vi "Pull_Data_via_Public_Client.vi"(3 "application reference":refnum<vi>, 4 "error in (no error)":errorcluster, 5 "Archive Files?":bool, 6 "Running on Server?":bool, 7 "Path of File relative to EnFlo Data Root":path[](array[path])) -> (0 "error out":errorcluster, 1 "Error String":string)   [LabVIEW 2016]
uses:
  Anemometry/Anemometry Sub Vis/Globals/Constants_global.vi
  Sub VIs/Harvest_Global.vi
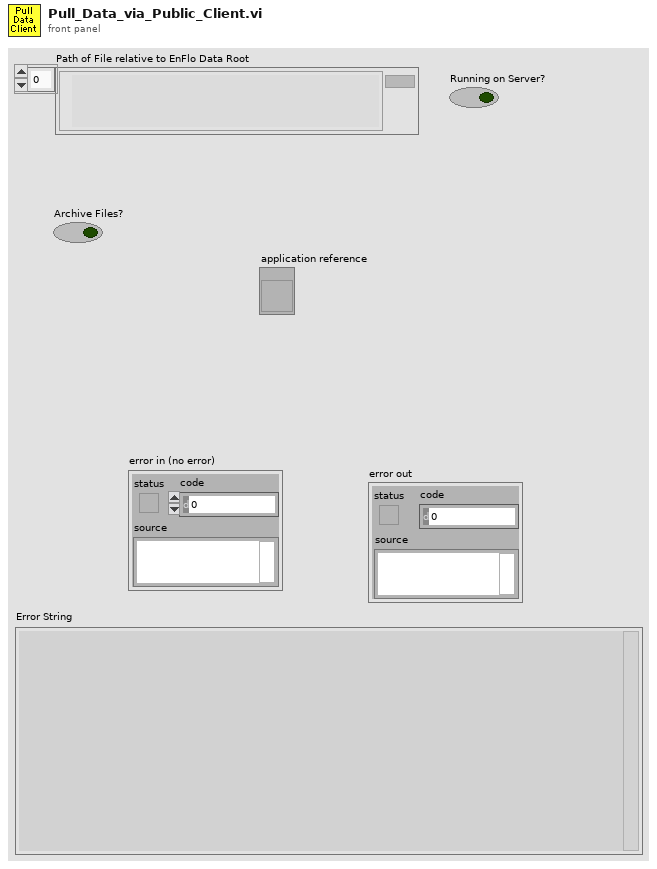
[diagram p1: front panel]
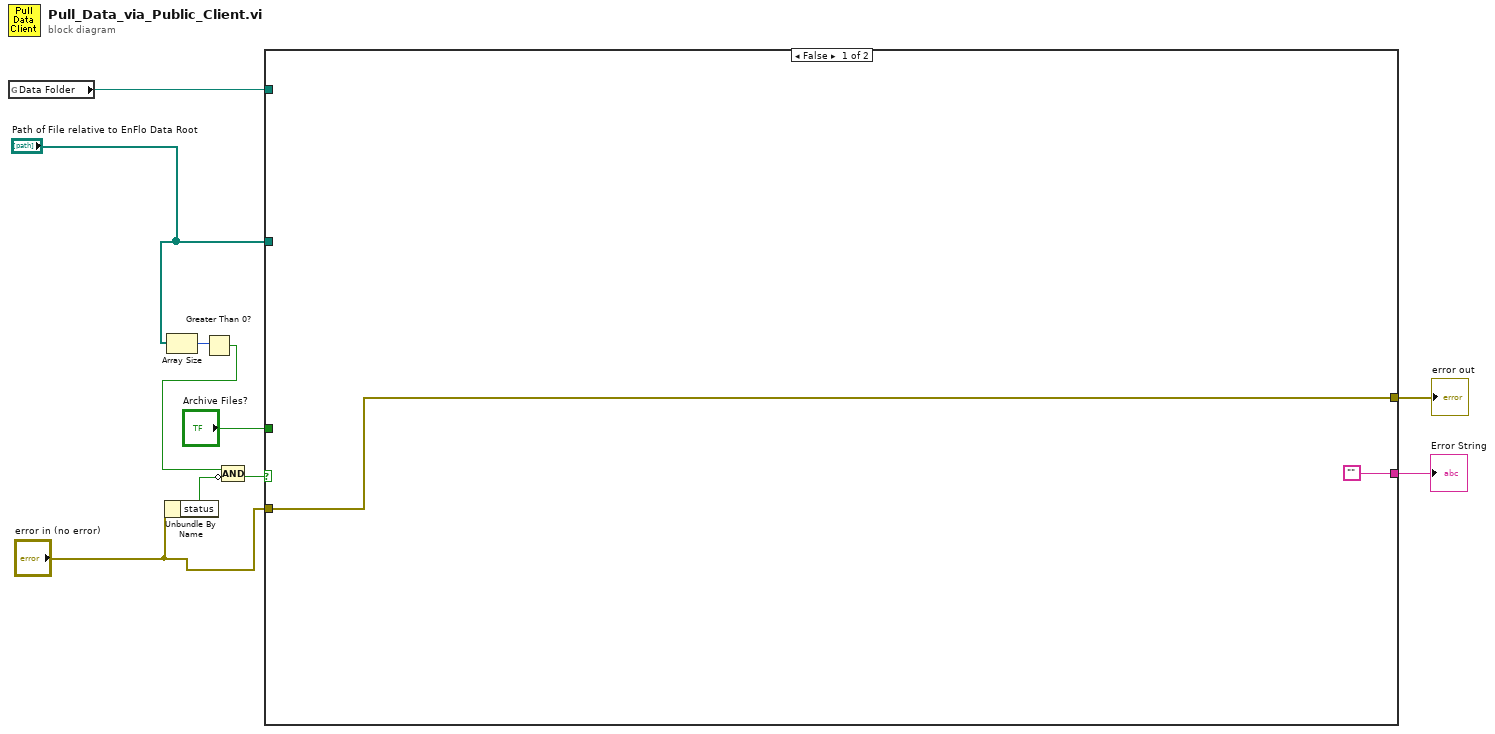
[diagram p0: block diagram]
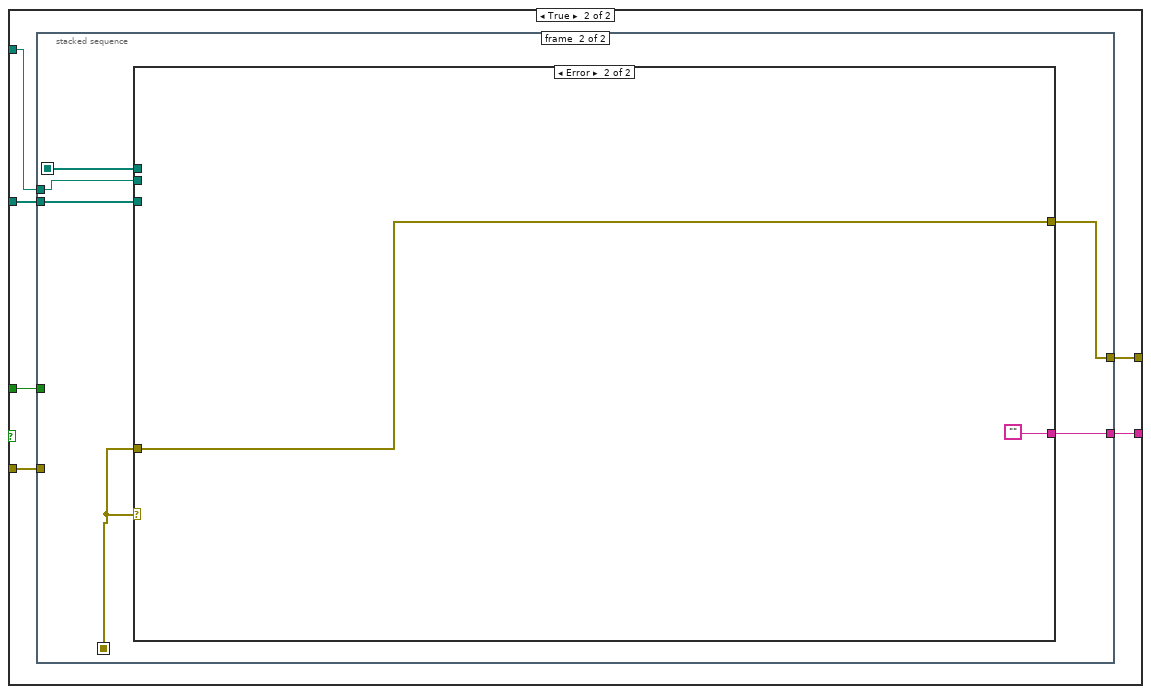
[diagram p2: hidden frame]
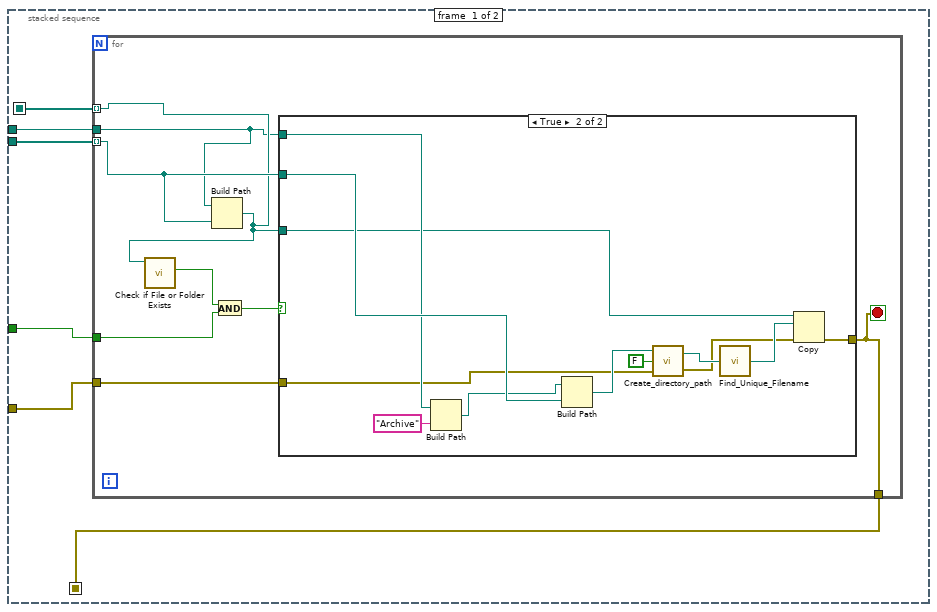
[diagram p3: hidden frame]
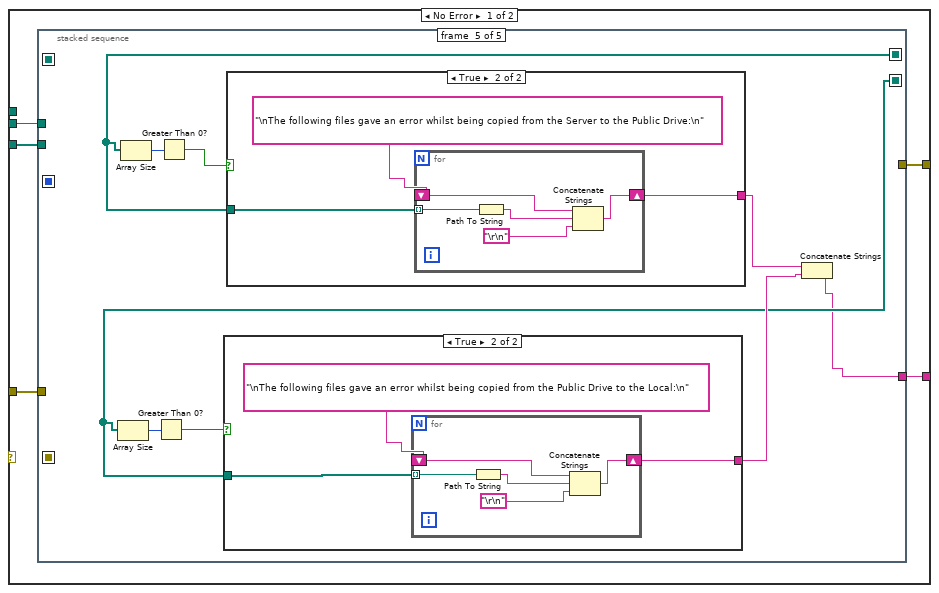
[diagram p5: hidden frame]
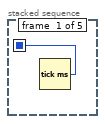
[diagram p6: hidden frame]
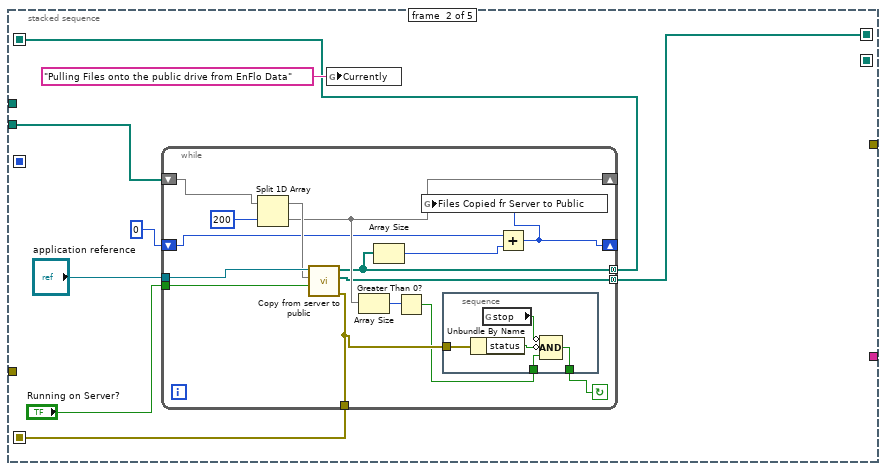
[diagram p7: hidden frame]
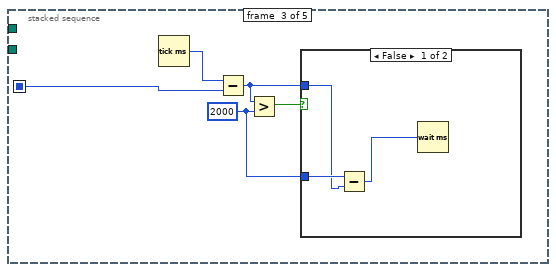
[diagram p8: hidden frame]
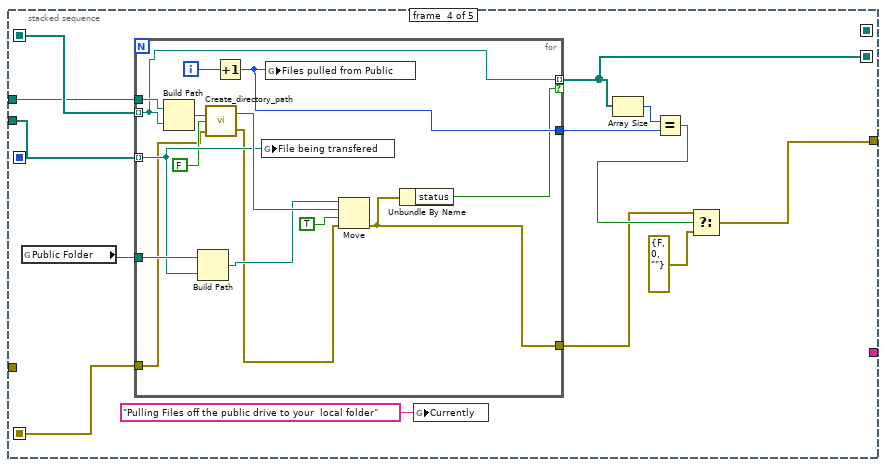
[diagram p10: hidden frame]
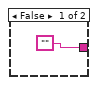
[diagram p11: hidden frame]
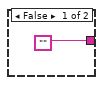
[diagram p12: hidden frame]
diagram:
  n1 = global read "Constants_global.vi" "Data Folder"() -> (w8:path)
  n2 = Unbundle By Name("error in (no error)") -> ("status"=w7:bool)
  n3 = Array Size(array="Path of File relative to EnFlo Data Root") -> (size(s)=w6:i32)
  n4 = Greater Than 0?(x=w6) -> (x > 0?=w5:bool)
  n5 = Compound Arithmetic op=AND(w5, invert w7) -> (w3:bool)
  n6 = case shown="False" w3 {
    tunnel: [w12 w18] -> w10
    tunnel: "error in (no error)" -> [w12 w17]
    tunnel: "Path of File relative to EnFlo Data Root" -> [_ w16]
    tunnel: "Archive Files?" -> [_ w15]
    tunnel: w8 -> [_ w14]
    tunnel: ["" w13] -> w1
    frame False {
    }
    frame True {
      n7 = stacked-sequence {
        seq-local: [w23 _] -> [_ w48]
        seq-local: [w21 _] -> [_ w50]
        tunnel: [_ w51] -> w18
        tunnel: w17 -> [w24 _]
        tunnel: w16 -> [w22 w49]
        tunnel: w15 -> [w20 _]
        tunnel: w14 -> [w19 w47]
        tunnel: [_ w46] -> w13
        frame #0 {
          n8 = for {
            tunnel: w24 -> [w32]
            tunnel: [w27] -> w23
            tunnel: w22 -> [w31] mode=indexing
            tunnel: w20 -> [w30]
            tunnel: [w26] -> w21 mode=indexing
            tunnel: w19 -> [w25]
            stop <- w27 stop-if-true
            n9 = Build Path(base path=w25, name or relative path=w31) -> (appended path=w26:path)
            n10 = call <vilib>:"Check if File or Folder Exists.vi"("path"=w26) -> ("file or folder exists?"=w29:bool)  [unwired: 8 in, 2 out]
            n11 = And(x=w29, y=w30) -> (x .and. y?=w28:bool)
            n12 = case shown="True" w28 {
              tunnel: w25 -> [_ w39]
              tunnel: w31 -> [_ w41]
              tunnel: [w33 w37] -> w27
              tunnel: w32 -> [w33 w36]
              tunnel: w26 -> [_ w35]
              frame False {
              }
              frame True {
                n13 = Build Path(base path=w39, name or relative path="Archive") -> (appended path=w38:path)
                n14 = Build Path(base path=w38, name or relative path=w41) -> (appended path=w44:path)
                n15 = call "Create_directory_path.vi"("error in (no error)"=w36, "Dialog Box"=FALSE, "Path name"=w44) -> ("error out"=w42:errorcluster, "Path name Out"=w43:path)
                n16 = call "Find_Unique_Filename.vi"("Path In"=w43) -> ("Unique Path Out"=w45:path)  [unwired: 2 in]
                n17 = Copy(8:w42, 10:w45, 11:w35) -> (0:w37:errorcluster)  [unwired: 2 in, 2 out]
              }
            }
          }
        }
        frame #1 {
          n18 = case shown="Error" w48 {
            tunnel: [w54 w150] -> w51
            tunnel: w48 -> [w55 w150]
            tunnel: w50 -> [_ _]
            tunnel: w49 -> [w56 _]
            tunnel: w47 -> [w53 _]
            tunnel: [w52 ""] -> w46
            frame No Error {
              n19 = stacked-sequence {
                seq-local: [_ w60 _ _ _] -> [_ _ _ w106 _]
                seq-local: [_ w64 _ _ _] -> [_ _ _ w103 _]
                seq-local: [w57 _ _ _ _] -> [_ _ w86 _ _]
                seq-local: [_ w58 _ _ _] -> [_ _ _ _ w124]
                seq-local: [_ _ _ w94 _] -> [_ _ _ _ w123]
                tunnel: w56 -> [_ w65 _ w104 _]
                tunnel: w55 -> [_ _ _ _ _]
                tunnel: [_ _ _ w95 _] -> w54
                tunnel: w53 -> [_ _ _ w102 _]
                tunnel: [_ _ _ _ w122] -> w52
                frame #0 {
                  n20 = Tick Count (ms)() -> (millisecond timer value=w57:u32)
                }
                frame #1 {
                  n21 = while {
                    tunnel: [w75] -> w64
                    tunnel: "application reference" -> [w80]
                    tunnel: "Running on Server?" -> [w79]
                    shift-right: [w73] -> _
                    shift-left: w65 -> [w77]
                    tunnel: [w70] -> w60 mode=concatenating
                    shift-right: [w67] -> _
                    shift-left: 0 -> [w68]
                    tunnel: [w66] -> w58 mode=concatenating
                    stop <- w71 continue-if-true
                    n22 = Split 1D Array(array=w77, index=200) -> (first subarray=w76:path[], second subarray=w73:path[])
                    n23 = call "Copy from server to public.vi"("Running on Server?"=w79, "Path of File relative to EnFlo Data Root"=w76, "Application in"=w80) -> ("error out"=w75:errorcluster, "Problem Files"=w66:path[], "Relative Paths Out"=w70:path[])  [unwired: 6 in]
                    n24 = Array Size(array=w73) -> (size(s)=w74:i32)
                    n25 = Array Size(array=w70) -> (size(s)=w69:i32)
                    n26 = Greater Than 0?(x=w74) -> (x > 0?=w72:bool)
                    n27 = stacked-sequence {
                      tunnel: [w84] -> w71
                      tunnel: w75 -> [w82]
                      tunnel: w72 -> [w81]
                      frame #0 {
                        n28 = Unbundle By Name(w82) -> ("status"=w85:bool)
                        n29 = global read "Harvest_Global.vi" "stop"() -> (w83:bool)
                        n30 = Compound Arithmetic op=AND(invert w83, invert w85, w81) -> (w84:bool)
                      }
                    }
                    n31 = Add(x=w68, y=w69) -> (x+y=w67:i32)
                    n32 = global write "Harvest_Global.vi" "Files Copied fr Server to Public"(w67) -> ()
                  }
                  n33 = global write "Harvest_Global.vi" "Currently"("Pulling Files onto the public drive from EnFlo Data" ("Currently Running")) -> ()
                }
                frame #2 {
                  w89 = u32 2000 ("y")
                  n34 = Tick Count (ms)() -> (millisecond timer value=w87:u32)
                  n35 = Subtract(x=w87, y=w86) -> (x-y=w90:u32)
                  n36 = Greater?(x=w90, y=w89) -> (0:w88:bool)
                  n37 = case shown="False" w88 {
                    tunnel: w89 -> [w93 _]
                    tunnel: w90 -> [w92 _]
                    frame False {
                      n38 = Subtract(x=w93, y=w92) -> (x-y=w91:u32)
                      n39 = Wait (ms)(milliseconds to wait=w91) -> ()  [unwired: 1 out]
                    }
                    frame True {
                    }
                  }
                }
                frame #3 {
                  n40 = global read "Constants_global.vi" "Public Folder"() -> (w105:path)
                  n41 = for {
                    tunnel: w106 -> [w109] mode=indexing
                    tunnel: w105 -> [w120]
                    tunnel: w104 -> [w114] mode=indexing
                    tunnel: w103 -> [w112]
                    tunnel: [w118] -> w96
                    tunnel: w102 -> [w116]
                    tunnel: [w110] -> w99
                    tunnel: [w109] -> w94 mode=indexing if=w107
                    i -> [w115]
                    n42 = Build Path(base path=w116, name or relative path=w109) -> (appended path=w117:path)
                    n43 = Build Path(base path=w120, name or relative path=w114) -> (appended path=w119:path)
                    n44 = call "Create_directory_path.vi"("error in (no error)"=w112, "Dialog Box"=FALSE, "Path name"=w117) -> ("error out"=w111:errorcluster, "Path name Out"=w121:path)
                    n45 = Increment(x=w115) -> (x+1=w110:i32)
                    n46 = global write "Harvest_Global.vi" "File being transfered"(w114) -> ()
                    n47 = global write "Harvest_Global.vi" "Files pulled from Public"(w110) -> ()
                    n48 = Move(source path=w119, error in=w111, 9:TRUE ("overwrite (F)"), 10:w121) -> (error out=w118:errorcluster)  [unwired: 1 in, 2 out]
                    n49 = Unbundle By Name(w118) -> ("status"=w107:bool)
                  }
                  n50 = global write "Harvest_Global.vi" "Currently"("Pulling Files off the public drive to your  local folder" ("Currently Running")) -> ()
                  n51 = Array Size(array=w94) -> (size(s)=w100:i32)
                  n52 = Equal?(x=w100, y=w99) -> (x = y?=w97:bool)
                  n53 = Select(t=w96, s=w97, f=errorcluster {"status"=FALSE, "code"=0, "source"=""} ("error out")) -> (s? t:f=w95:errorcluster)
                }
                frame #4 {
                  n54 = Array Size(array=w123) -> (size(s)=w128:i32)
                  n55 = Array Size(array=w124) -> (size(s)=w125:i32)
                  n56 = Greater Than 0?(x=w128) -> (x > 0?=w127:bool)
                  n57 = Greater Than 0?(x=w125) -> (x > 0?=w126:bool)
                  n58 = case shown="True" w127 {
                    tunnel: w123 -> [_ w134]
                    tunnel: ["" w132] -> w130
                    frame False {
                    }
                    frame True {
                      n59 = for {
                        tunnel: w134 -> [w139] mode=indexing
                        shift-right: [w136] -> w132
                        shift-left: "\nThe following files gave an error whilst being copied from the Public Drive to the Local:\n" -> [w135]
                        n60 = Path To String(path=w139) -> (string=w138:string)
                        n61 = Concatenate Strings(w135, w138, "\r\n") -> (w136:string)
                      }
                    }
                  }
                  n62 = case shown="True" w126 {
                    tunnel: w124 -> [_ w143]
                    tunnel: ["" w141] -> w129
                    frame False {
                    }
                    frame True {
                      n63 = for {
                        tunnel: w143 -> [w148] mode=indexing
                        shift-right: [w145] -> w141
                        shift-left: "\nThe following files gave an error whilst being copied from the Server to the Public Drive:\n" -> [w144]
                        n64 = Path To String(path=w148) -> (string=w147:string)
                        n65 = Concatenate Strings(w144, w147, "\r\n") -> (w145:string)
                      }
                    }
                  }
                  n66 = Concatenate Strings(w129, w130) -> (w122:string)
                }
              }
            }
            frame Error {
            }
          }
        }
      }
    }
  }
  "error out" <- w10
  "Error String" <- w1
